vi "Configure Measurement Auto Range Upper Limit.vi"(8 "error in (no error)":errorcluster, 9 "Upper Limit (0.2)":dbl=0.2, 10 "Function (0: Resistance)":u16(ring) items=["Resistance"], 11 "VISA resource name":refnum<visa-resource-name>) -> (0 "error out":errorcluster, 3 "VISA resource name out":refnum<visa-resource-name>)   [LabVIEW 2015, in "Keithley 2450.lvlib"]
doc: "When autorange is selected, this VI selects the upper limit for measurements of the selected function."
uses:
  <instrlib>/Keithley 2450/Keithley 2450.lvlib
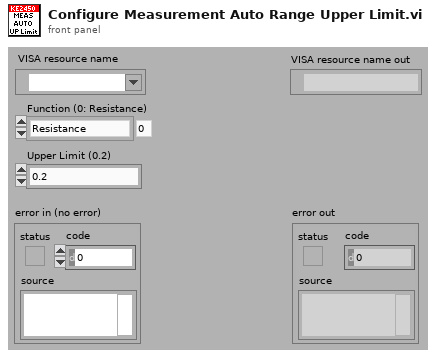
[diagram p1: front panel]
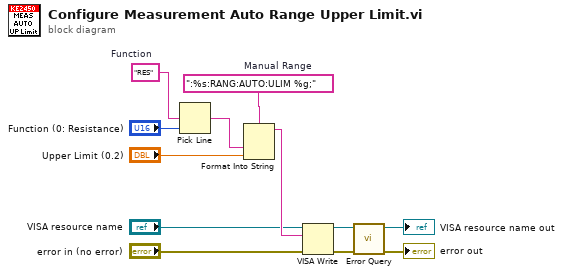
[diagram p0: block diagram]
diagram:
  w7 = "RES"  # Function
  w9 = ":%s:RANG:AUTO:ULIM %g;"  # Manual Range
  n1 = Pick Line(multi-line string=w7, line index="Function (0: Resistance)") -> (output string=w5:string)  [unwired: 1 out]
  n2 = Format Into String(format string=w9, w5, "Upper Limit (0.2)") -> (resulting string=w10:string)  [unwired: 2 in, 1 out]
  n3 = VISA Write(VISA resource name="VISA resource name", write buffer=w10, error in (no error)="error in (no error)") -> (VISA resource name out=w4:refnum<visa-resource-name>, error out=w3:errorcluster)  [unwired: 1 out]
  n4 = call <instrlib>:"Error Query.vi"("error in (no error)"=w3, "VISA resource name"=w4) -> ("error out"=→"error out":errorcluster, "VISA resource name out"=→"VISA resource name out":refnum<visa-resource-name>)  [unwired: 8 out]
